vi "Stop Core.vi"(10 "final error code":i32, 11 "startconteo in":refnum<class "startconteo.lvclass">) -> (3 "startconteo out":refnum<class "startconteo.lvclass">)   [LabVIEW 2019, in "startconteo.lvlib" / "startconteo.lvclass"]
doc: "(<B>Filename</B>: Actor Framework.lvlib:Actor.lvclass:Stop Core.vi)\n\nDefines what the actor does before it stops. Use the <B>final error code</B> input to determine whether the actor shut down in response to an error.\n\nBy default, this method passes the Stop message along to all auto-stop nested actors. A descendant class may override this method to define additional behavior, such as shutting down any processes the actor initiated in its override of the Actor Core method."
uses:
  startconteo.lvclass
  <vilib>/ActorFramework/Actor/Actor.lvclass
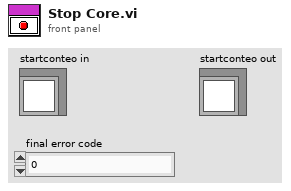
[diagram p1: front panel]
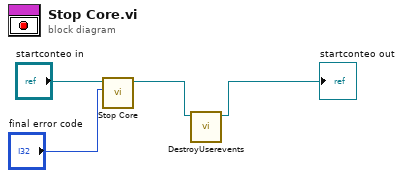
[diagram p0: block diagram]
diagram:
  n1 = call-parent "Stop Core.vi"("final error code"="final error code", "Actor in"="startconteo in") -> ("Actor out"=w2:refnum<class "startconteo.lvclass">)  [unwired: 9 in]
  n2 = call "DestroyUserevents.vi"("startconteo in"=w2) -> ("startconteo out"=→"startconteo out":refnum<class "startconteo.lvclass">)  [unwired: 9 in, 1 out]
